vi "Com_SECS Equipment _Session Write.vi"(8 "error in":errorcluster, 9 "Timeout(100)":i32=100, 10 "Write Data":string, 11 "Session In":refnum<k5>) -> (0 "error out":errorcluster, 3 "Session Out":refnum<k5>)   [LabVIEW 2016]
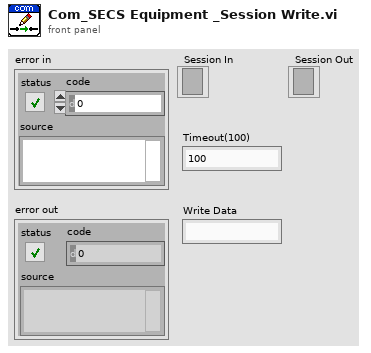
[diagram p1: front panel]
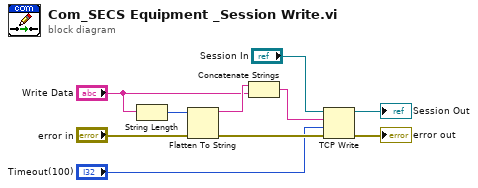
[diagram p0: block diagram]
diagram:
  n1 = String Length(string="Write Data") -> (length=w10:i32)
  n2 = Flatten To String(anything=w10, error in (no error)="error in") -> (data string=w9:string, error out=w7:errorcluster)  [unwired: 3 out]
  n3 = Concatenate Strings(w9, "Write Data") -> (w8:string)
  n4 = TCP Write(connection ID="Session In", data in=w8, error in (no error)=w7, 9:"Timeout(100)") -> (connection ID out=→"Session Out":refnum<k5>, error out=→"error out":errorcluster)  [unwired: 1 out]
